vi "Prep Alarm Tags.vi"(11 "Alarm Tag Description path":path) -> (2 "Alarm Array":T1[](array[typedef]), 3 "CVT Tags to Create":T5)   [LabVIEW 2019]
uses:
  <vilib>/NI/Current Value Table/Type Defs/File Format.ctl
  <vilib>/NI/Current Value Table/Type Defs/Single Tag.ctl
  <vilib>/NI/Current Value Table/Type Defs/Data Types.ctl
  <vilib>/NI/Current Value Table/Type Defs/Tag Grouping set.ctl
  <userlib>/TAE/_SubVIs/TypeDefs/tae_AlarmTagConfiguration.ctl
  <vilib>/NI/Current Value Table/Compatibility/_SubVIs/TypeDefs/cvt_Data Types.ctl
  <userlib>/TAE/_SubVIs/TypeDefs/tae_AlarmConfiguration.ctl
  <userlib>/TAE/_SubVIs/TypeDefs/tae_AlarmType.ctl
  <vilib>/NI/Current Value Table/Current Value Table.lvlib
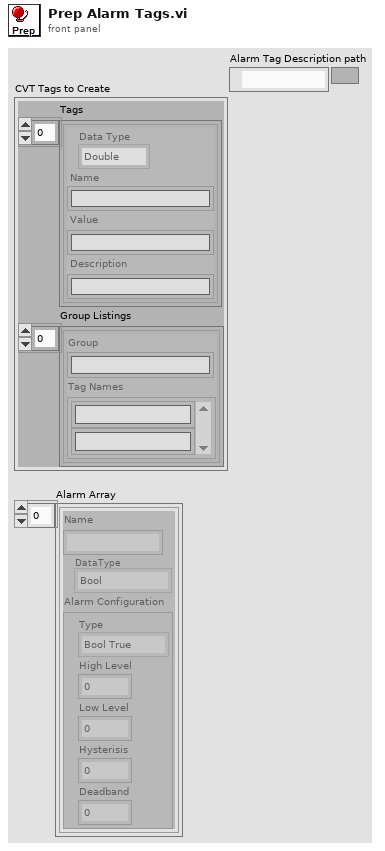
[diagram p1: front panel]
types:
  T1 = typedef "tae_AlarmTagConfiguration.ctl" = cluster{"Name":string, "DataType":T2, "Alarm Configuration":T3}
  T2 = typedef "cvt_Data Types.ctl" = enum16{"Bool", "U8", "I32", "Double", "String", "Enum"}
  T3 = typedef "tae_AlarmConfiguration.ctl" = cluster{"Type":T4, "High Level":dbl, "Low Level":dbl, "Hysterisis":dbl, "Deadband":dbl}
  T4 = typedef "tae_AlarmType.ctl" = enum32{"Bool True", "Bool False", "Over Limit", "Under Limit", "Out-of-Range", "Enum Equal", "Enum Not Equal"}
  T5 = typedef "Current Value Table.lvlib/File Format.ctl" = cluster{"Tags":T6[], "Group Listings":T8[]}
  T6 = typedef "Current Value Table.lvlib/Single Tag.ctl" = cluster{"Data Type":T7, "Name":string, "Value":string, "Description":string}
  T7 = typedef "Current Value Table.lvlib/Data Types.ctl" = enum16{"Double", "Single", "I64", "I32", "I16", "I8", "U64", "U32", "U16", "U8", "String", "Boolean", "Array of U8", "Array of U16", "Array of U32", "Array of U64", "Array of I64", "Array of I32", "Array of I16", "Array of I8", "Array of Double", "Array of Single", "Array of Boolean", "Array of String"}
  T8 = typedef "Current Value Table.lvlib/Tag Grouping set.ctl" = cluster{"Group":string, "Tag Names":string[]}
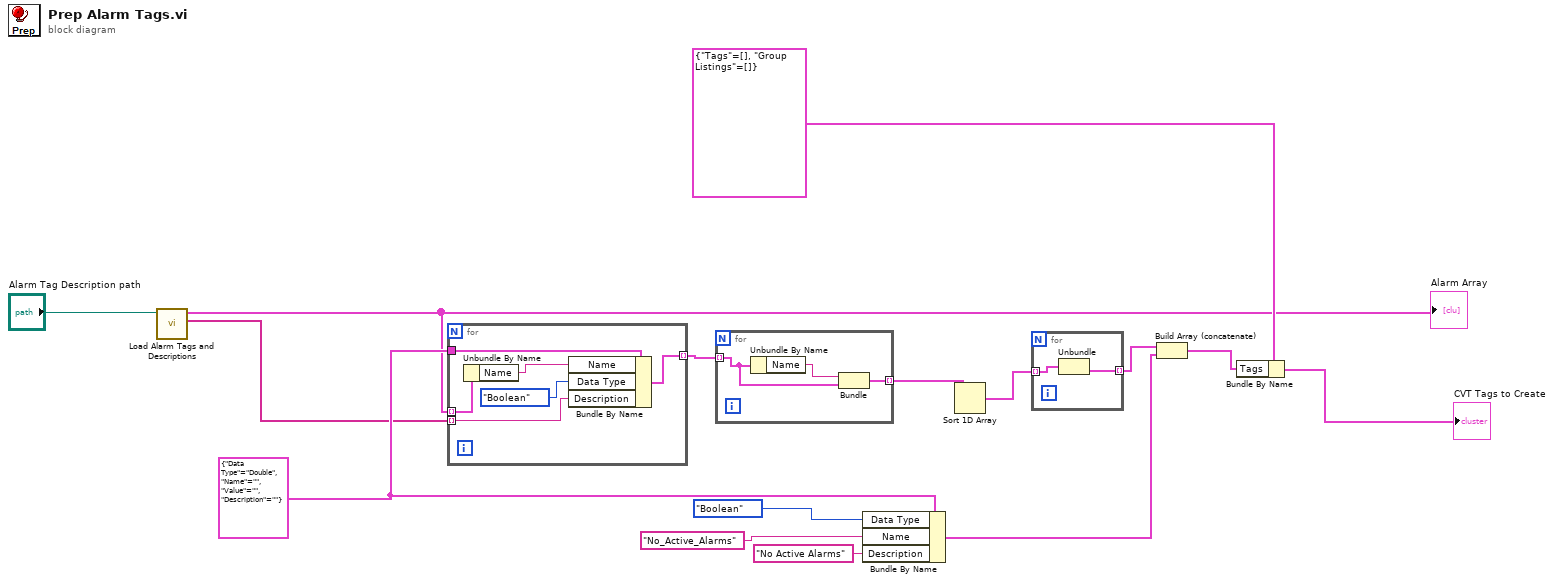
[diagram p0: block diagram]
diagram:
  w9 = T6 {"Data Type"=enum."Double", "Name"="", "Value"="", "Description"=""} ("Tag")
  n1 = call "Load Alarm Tags and Descriptions.vi"("Alarm Tag Description path"="Alarm Tag Description path") -> ("Alarm Descriptions"=w2:string[], "Alarm Array"=w5:T1[])  [unwired: 9 in]
  "Alarm Array" <- w5
  n2 = for {
    tunnel: w5 -> [w21] mode=indexing
    tunnel: w2 -> [w18] mode=indexing
    tunnel: [w19] -> w3 mode=indexing
    tunnel: w9 -> [w17]
    n3 = Unbundle By Name(w21) -> ("Name"=w20:string)
    n4 = Bundle By Name(cluster=w17, "Name"=w20, "Data Type"=Data_Types."Boolean", "Description"=w18) -> (w19:T6)
  }
  n5 = for {
    tunnel: w3 -> [w23] mode=indexing
    tunnel: [w22] -> w4 mode=indexing
    n6 = Unbundle By Name(w23) -> ("Name"=w24:string)
    n7 = Bundle("Name"=w24, "Tag"=w23) -> (w22:cluster{"Name":string, "Tag":T6})  [unwired: 1 in]
  }
  n8 = Bundle By Name(cluster=w9, "Data Type"=Data_Types."Boolean", "Name"="No_Active_Alarms" ("All Languages"), "Description"="No Active Alarms") -> (w14:T6)
  n9 = Sort 1D Array(array=w4) -> (sorted array=w7:cluster{"Name":string, "Tag":T6}[])
  n10 = for {
    tunnel: w7 -> [w26] mode=indexing
    tunnel: [w25] -> w13 mode=indexing
    n11 = Unbundle(w26) -> ("Tag"=w25:T6)  [unwired: 1 out]
  }
  n12 = Build Array (concatenate)(w13, w14) -> (w15:T6[])
  n13 = Bundle By Name(cluster=T5 {"Tags"=[], "Group Listings"=[]} ("CVT Tags to Create"), "Tags"=w15) -> (→"CVT Tags to Create":T5)
